vi "Call Interface.vi"() -> (0 "UserMessage":refnum<user-event>, 1 "UUT Result":refnum<user-event>, 2 "exit":refnum<user-event>, 3 "ref":refnum<notifier>)   [LabVIEW 2025, in "Test Unit.lvlib"]
uses:
  Test Unit.lvlib
  UUT Result.ctl
  <vilib>/Test Bench Framework/Test Executive.lvlibp/TestEngine/TestEngine/TestEngine/Typedefs/Report General.ctl
  Full User Interface/Send User Message Argument--cluster.ctl
  Interface.vi
  <vilib>/Test Bench Framework/Test Executive.lvlibp/TestEngine/TestEngine/TestEngine/Test Engine.lvclass
  Full User Interface/Full User Interface.lvlib
panel:
  out "error out":errorcluster
  in  "error in (no error)":errorcluster
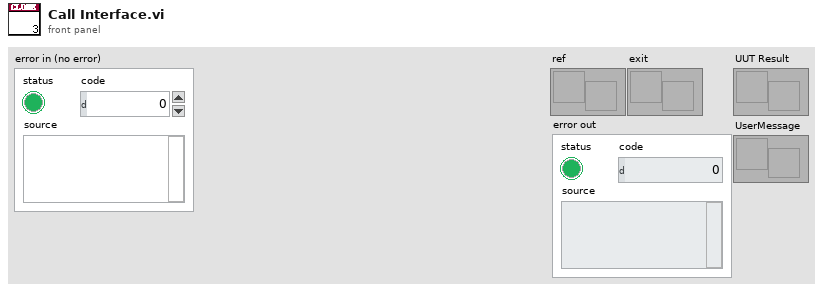
[diagram p1: front panel]
types:
  T1 = typedef "Full User Interface.lvlib/Send User Message Argument--cluster.ctl" = cluster{"Station ID":i32, "Socket":i32, "UserMessage":string, "MessageData":variant}
  T2 = typedef "Test Unit.lvlib/UUT Result.ctl" = cluster{"Station":i32, "Socket":i32, "DetailTestResult":string[][], "Report Path":path, "General":T3}
  T3 = typedef "Test Executive.lvlibp/Test Engine.lvlib/Test Engine.lvclass/Report General.ctl" = cluster{"Sequence Path":path, "Serial Number":string, "Test Date Time":timestamp, "UUT Status":string, "Faulty Item":string, "Seconds Executing":dbl}
  T4 = cluster{"UUT State":refnum<vi>, "Cycle Time":refnum<vi>, "SerialNumber":refnum<vi>, "Tree":refnum<vi>, "This VI":refnum<vi>}
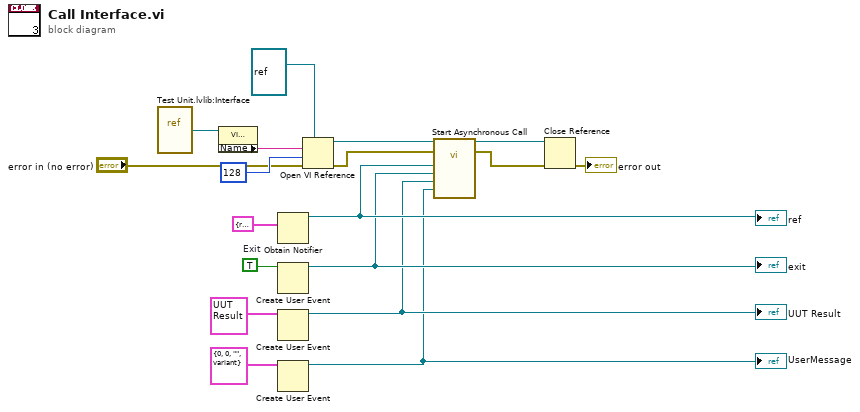
[diagram p0: block diagram]
diagram:
  w11 = TRUE  # Exit
  n1 = vi-ref "Test Unit.lvlib:Interface.vi"() -> (w18:refnum<vi>)
  n2 = property class="VI (strict)"(reference=w18) -> ("Name"=w17:string)  [unwired: 1 in, 2 out]
  n3 = Obtain Notifier(notification data type=T4 {"UUT State"=refnum, "Cycle Time"=refnum, "SerialNumber"=refnum, "Tree"=refnum, "This VI"=refnum} ("output cluster")) -> (notifier out=w9:refnum<notifier>)  [unwired: 3 in, 2 out]
  "ref" <- w9
  n4 = Create User Event(user event datatype=w11) -> (user event=w8:refnum<user-event>)  [unwired: 1 in, 1 out]
  "exit" <- w8
  n5 = Create User Event(user event datatype=T2 {"Station"=0, "Socket"=0, "DetailTestResult"=[], "Report Path"=path "", "General"={"Sequence Path"=path "", "Serial Number"="", "Test Date Time"=timestamp(0 s since 1904-01-01), "UUT Status"="", "Faulty Item"="", "Seconds Executing"=0.0}} ("output cluster")) -> (user event=w4:refnum<user-event>)  [unwired: 1 in, 1 out]
  "UUT Result" <- w4
  n6 = Create User Event(user event datatype=T1 {"Station ID"=0, "Socket"=0, "UserMessage"="", "MessageData"=variant(cluster{"Socket":i32, "UserMessage":string, "MessageData":variant} {"Socket"=0, "UserMessage"="", "MessageData"=variant})} ("DQMH_ARG")) -> (user event=w1:refnum<user-event>)  [unwired: 1 in, 1 out]
  "UserMessage" <- w1
  n7 = Open VI Reference(type specifier VI Refnum (for type only)=refnum<vi> refnum, vi path=w17, options=128, error in (no error)="error in (no error)") -> (vi reference=w15:refnum<vi>, error out=w13:errorcluster)  [unwired: 2 in]
  n8 = call-by-ref "Start Asynchronous Call"(reference=w15, error in=w13, "UserMessage"=w1, "UUT Result"=w4, "Exit"=w8, "VI ref"=w9) -> (reference out=w14:refnum<vi>, error out=w12:errorcluster)  [unwired: 8 in]
  n9 = Close Reference(reference=w14, error in (no error)=w12) -> (error out=→"error out":errorcluster)
